vi "aFGV - Read Write Config RT.vi"(6 "State":enum16{"Read", "Write", "Delete"}(ring), 7 "Section":T1=enum."Acquisition Setting", 8 "Error In":errorcluster, 9 "File name":string, 10 "Key Name":string, 11 "Data in":string[](array[string])) -> (0 "Error Out":errorcluster, 2 "Data out":string[](array[string]), 3 "Key Names":string[](array[string]))   [LabVIEW 2020]
uses:
  Control/Section Config RT.ctl
  Control/FGV State.ctl
  <vilib>/Utility/config.llb/Read Key (String).vi
  <vilib>/Utility/config.llb/Write Key (String).vi
  <vilib>/Utility/config.llb/NI_LVConfig.lvlib
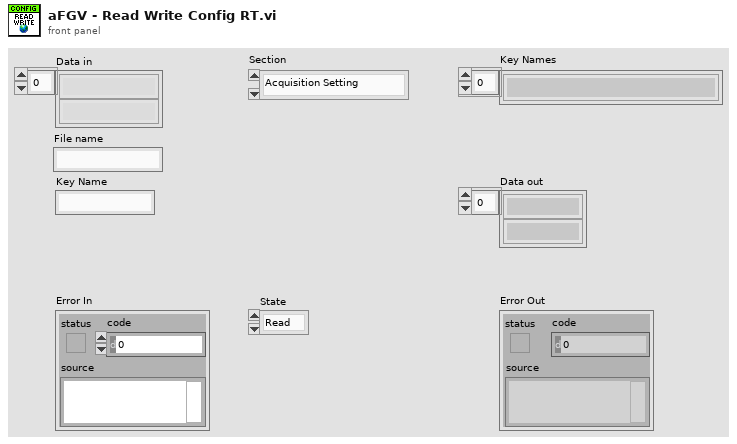
[diagram p1: front panel]
types:
  T1 = typedef "Section Config RT.ctl" = enum16{"Mod1/AI0", "Mod1/AI1", "Mod1/AI2", "Mod1/AI3", "Network Stream", "Acquisition Setting"}
  T2 = typedef "FGV State.ctl" = enum16{"Write", "Read"}
  T3 = typedef "NI_LVConfig.lvlib/Config Data RefNum.ctl" = refnum<k1>
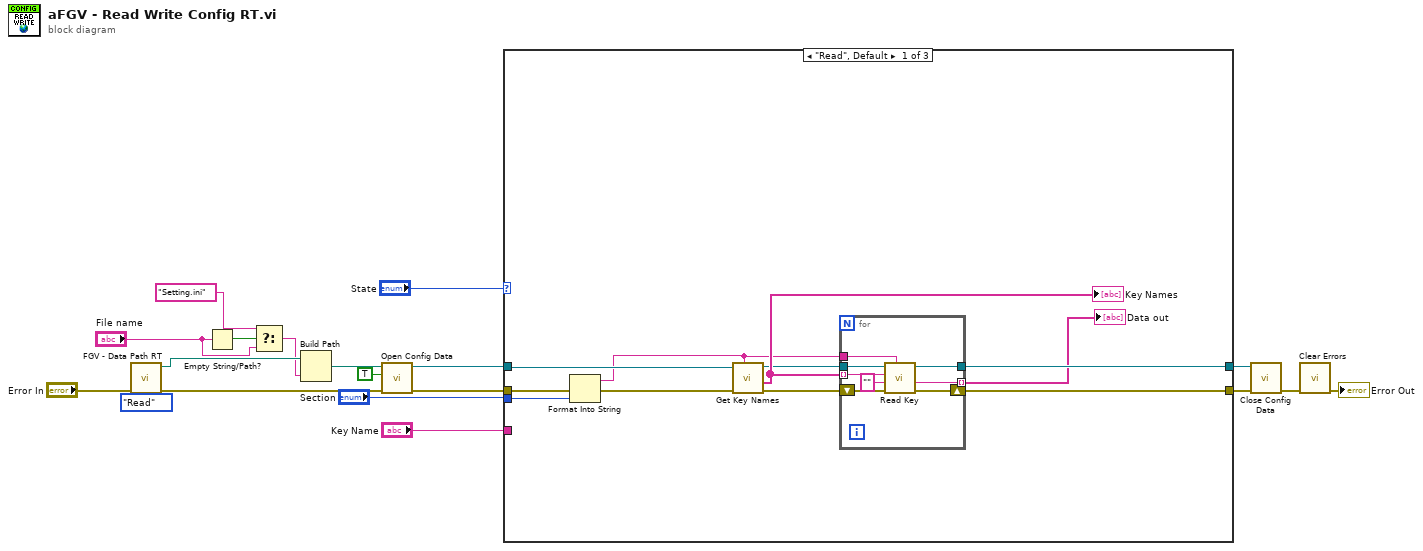
[diagram p0: block diagram]
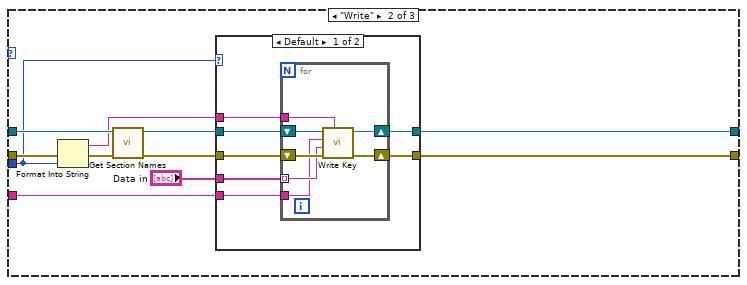
[diagram p2: hidden frame]
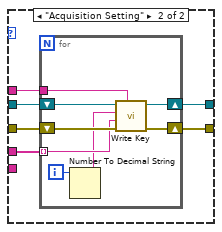
[diagram p3: hidden frame]
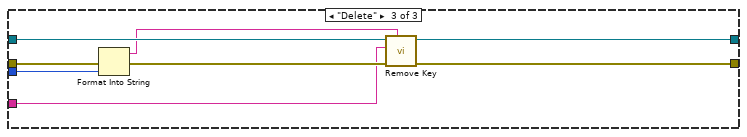
[diagram p4: hidden frame]
diagram:
  n1 = call "FGV - Data Path RT.vi"("FGV State"=FGV_State."Read", "Error In"="Error In") -> ("Error Out"=w14:errorcluster, "Path Out"=w7:path)  [unwired: 8 in]
  n2 = Empty String/Path?(string/path="File name") -> (empty?=w2:bool)
  n3 = Select(t="Setting.ini" ("name or relative path"), s=w2, f="File name") -> (s? t:f=w3:string)
  n4 = Build Path(base path=w7, name or relative path=w3) -> (appended path=w11:path)
  n5 = call <vilib>:"Open Config Data.vi"("error in (no error)"=w14, "create file if necessary (T)"=TRUE, "configuration file path"=w11) -> ("error out"=w19:errorcluster, "refnum"=w13:T3)  [unwired: 6 in, 1 out]
  n6 = case shown="\"Read\", Default" "State" {
    tunnel: w19 -> [w28 w49 w85]
    tunnel: w13 -> [w27 w45 w82]
    tunnel: [w30 w48 w84] -> w18
    tunnel: [w26 w44 w80] -> w12
    tunnel: "Section" -> [w23 w40 w79]
    tunnel: "Key Name" -> [_ w41 w81]
    frame "Read", Default {
      n7 = Format Into String(error in=w28, w23) -> (resulting string=w20:string, error out=w29:errorcluster)  [unwired: 2 in]
      n8 = call <vilib>:"Get Key Names.vi"("section"=w20, "error in (no error)"=w29, "refnum"=w27) -> ("error out"=w22:errorcluster, "key names"=w25:string[], "refnum out"=w21:T3)  [unwired: 5 in, 1 out]
      "Key Names" <- w25
      n9 = for {
        tunnel: w21 -> [w36]
        shift-right: [w38] -> w30
        shift-left: w22 -> [w37]
        tunnel: w25 -> [w35] mode=indexing
        tunnel: [w33] -> w26
        tunnel: [w32] -> w24 mode=indexing
        tunnel: w20 -> [w31]
        n10 = call-poly <vilib>:"Read Key.vi"("section"=w31, "error in (no error)"=w37, "default value"="", "key"=w35, "refnum"=w36) -> ("error out"=w38:errorcluster, "value"=w32:string, "refnum out"=w33:T3)  [unwired: 3 in, 1 out]
      }
      "Data out" <- w24
    }
    frame "Write" {
      n11 = Format Into String(error in=w49, w40) -> (resulting string=w39:string, error out=w46:errorcluster)  [unwired: 2 in]
      n12 = call <vilib>:"Get Section Names.vi"("error in (no error)"=w46, "refnum"=w45) -> ("error out"=w47:errorcluster, "refnum out"=w43:T3)  [unwired: 7 in, 1 out]
      n13 = case shown="Default" w40 {
        tunnel: w47 -> [w56 w69]
        tunnel: [w55 w68] -> w48
        tunnel: w39 -> [w54 w67]
        tunnel: w43 -> [w53 w66]
        tunnel: [w52 w65] -> w44
        tunnel: "Data in" -> [w51 w64]
        tunnel: w41 -> [w50 _]
        frame Default {
          n14 = for {
            tunnel: w54 -> [w61]
            tunnel: w51 -> [w58] mode=indexing
            shift-right: [w62] -> w55
            shift-left: w56 -> [w63]
            shift-right: [w59] -> w52
            shift-left: w53 -> [w60]
            tunnel: w50 -> [w57]
            n15 = call-poly <vilib>:"Write Key.vi"("section"=w61, "error in (no error)"=w63, "value"=w58, "key"=w57, "refnum"=w60) -> ("error out"=w62:errorcluster, "refnum out"=w59:T3)  [unwired: 4 in, 1 out]
          }
        }
        frame "Acquisition Setting" {
          n16 = for {
            tunnel: w67 -> [w75]
            tunnel: w64 -> [w72] mode=indexing
            shift-right: [w76] -> w68
            shift-left: w69 -> [w77]
            shift-right: [w73] -> w65
            shift-left: w66 -> [w74]
            i -> [w71]
            n17 = Number To Decimal String(number=w71) -> (decimal integer string=w70:string)  [unwired: 1 in]
            n18 = call-poly <vilib>:"Write Key.vi"("section"=w75, "error in (no error)"=w77, "value"=w72, "key"=w70, "refnum"=w74) -> ("error out"=w76:errorcluster, "refnum out"=w73:T3)  [unwired: 4 in, 1 out]
          }
        }
      }
    }
    frame "Delete" {
      n19 = Format Into String(error in=w85, w79) -> (resulting string=w78:string, error out=w83:errorcluster)  [unwired: 2 in]
      n20 = call <vilib>:"Remove Key.vi"("section"=w78, "error in (no error)"=w83, "key"=w81, "refnum"=w82) -> ("error out"=w84:errorcluster, "refnum out"=w80:T3)  [unwired: 5 in, 1 out]
    }
  }
  n21 = call <vilib>:"Close Config Data.vi"("error in (no error)"=w18, "refnum"=w12) -> ("error out"=w17:errorcluster)  [unwired: 8 in, 1 out]
  n22 = call <vilib>:"Clear Errors.vi"("error in (no error)"=w17) -> ("error out"=→"Error Out":errorcluster)  [unwired: 5 in, 1 out]
